vi "ActionVIOnCompile.vi"(8 "error in (no error)":errorcluster, 11 "Device Item Ref in":T3 format="%.0x") -> (0 "error out":errorcluster)   [LabVIEW 2017]
uses:
  <vilib>/NI Veristand/Custom Device API/Custom Device Item Ref.ctl
  Shared/Constants.vi
  <vilib>/NI Veristand/Custom Device API/Get Item Property (I32).vi
  <vilib>/NI Veristand/Custom Device API/Get Item Property (U32).vi
  <vilib>/NI Veristand/Custom Device API/Get Item Property (String).vi
  <vilib>/NI Veristand/Custom Device API/Set Item Property (Variant).vi
  <vilib>/NI Veristand/Custom Device API/Custom Device API.lvlib
  Shared/O2SensorSim_SLSC Shared.lvlib
panel:
  in  "Compiled.Settings 2":T1={"Name"="", "SLSC IP Address"="", "Slot #"=0, "Configuration Data"={"Properties"={"Boolean Properties"=[], "Double Properties"=[], "I32 Properties"=[], "I64 Properties"=[], "String Properties"=[], "U32 Properties"=[], "U64 Properties"=[]}}, "SLSC Set Properties"=[], "SLSC Get Properties"=[], "SLSC Commands"=[], "Username"="admin", "Password"="", "Support Modules"=[]}
  out "Found":bool
  out "support module":T2(array[cluster])
  out "appended array 2":T2(array[cluster]) {"Dev.ProductNumber" format="%.0x"; "Dev.VendorNumber" format="%.0x"}
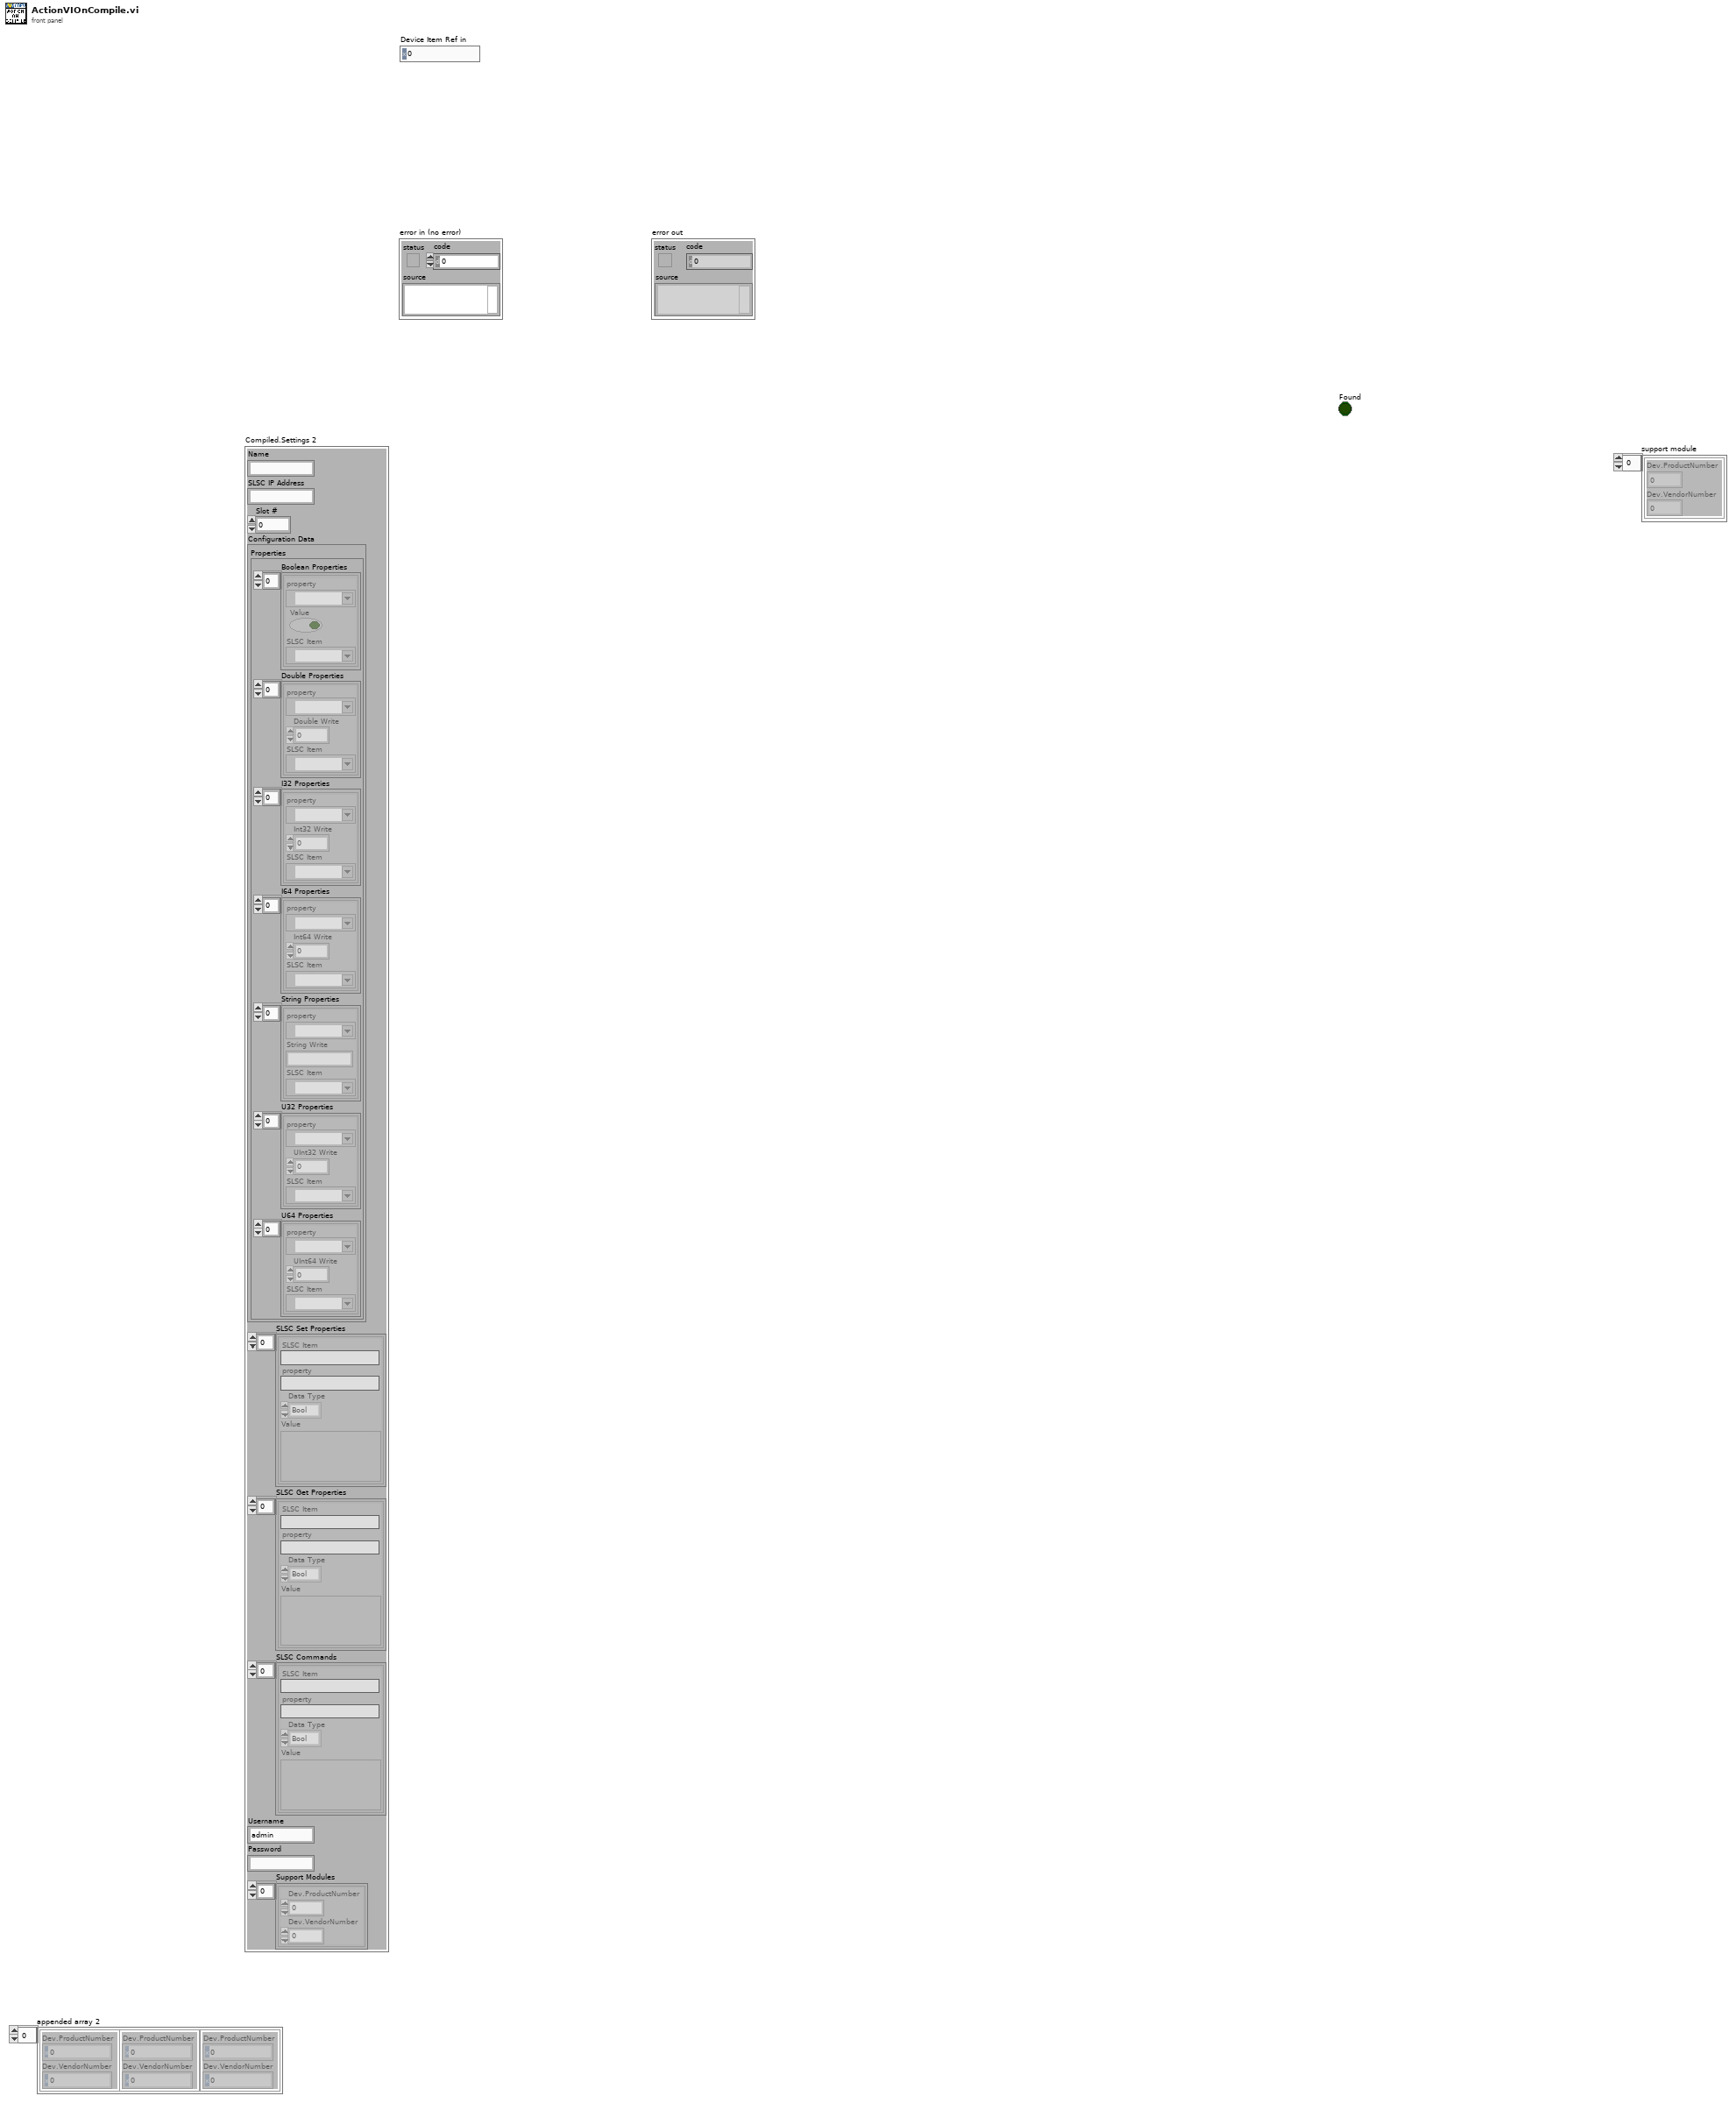
[diagram p1: front panel]
types:
  T1 = cluster{"Name":string, "SLSC IP Address":string, "Slot #":i32, "Configuration Data":cluster{"Properties":cluster{"Boolean Properties":cluster{"property":refnum<k21>, "Value":bool, "SLSC Item":refnum<k21>}[], "Double Properties":cluster{"property":refnum<k21>, "Double Write":dbl, "SLSC Item":refnum<k21>}[], "I32 Properties":cluster{"property":refnum<k21>, "Int32 Write":i32, "SLSC Item":refnum<k21>}[], "I64 Properties":cluster{"property":refnum<k21>, "Int64 Write":i64, "SLSC Item":refnum<k21>}[], "String Properties":cluster{"property":refnum<k21>, "String Write":string, "SLSC Item":refnum<k21>}[], "U32 Properties":cluster{"property":refnum<k21>, "UInt32 Write":u32, "SLSC Item":refnum<k21>}[], "U64 Properties":cluster{"property":refnum<k21>, "UInt64 Write":u64, "SLSC Item":refnum<k21>}[]}}, "SLSC Set Properties":cluster{"SLSC Item":string, "property":string, "Data Type":enum16{"Bool", "Double", "I32", "I64", "String", "U32", "U64", "EnumI32"}, "Value":variant}[], "SLSC Get Properties":cluster{"SLSC Item":string, "property":string, "Data Type":enum16{"Bool", "Double", "I32", "I64", "String", "U32", "U64", "EnumI32"}, "Value":variant}[], "SLSC Commands":cluster{"SLSC Item":string, "property":string, "Data Type":enum16{"Bool", "Double", "I32", "I64", "String", "U32", "U64", "EnumI32"}, "Value":variant}[], "Username":string, "Password":string, "Support Modules":cluster{"Dev.ProductNumber":u32, "Dev.VendorNumber":u32}[]}
  T2 = cluster{"Dev.ProductNumber":u32, "Dev.VendorNumber":u32}[]
  T3 = typedef "Custom Device API.lvlib/Custom Device Item Ref.ctl" = u64
  T4 = cluster{"Dev.ProductNumber":u32, "Dev.VendorNumber":u32}
  T5 = typedef "Custom Device API.lvlib/Custom Device Item Info.ctl" = cluster{"Name":string, "Is Channel":bool, "GUID":string, "Is Waveform":bool}
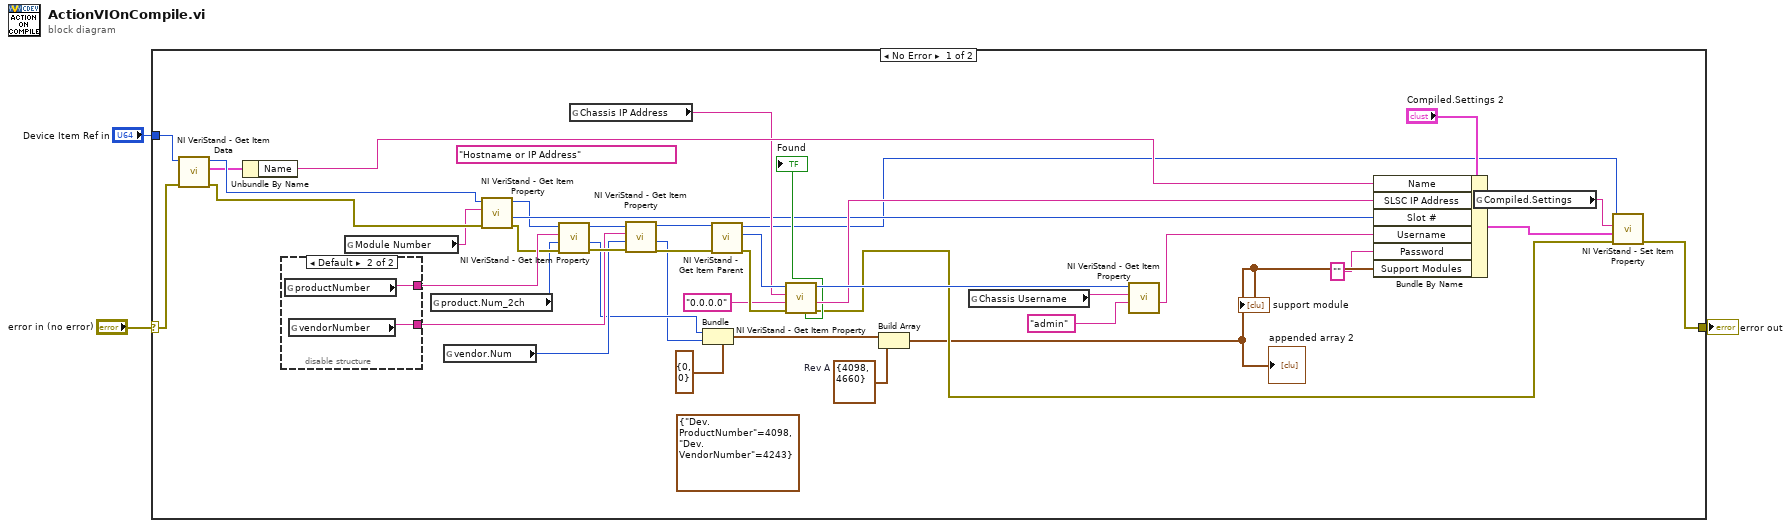
[diagram p0: block diagram]
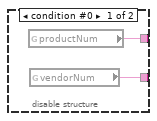
[diagram p2: hidden frame]
diagram:
  n1 = case shown="No Error" "error in (no error)" {
    selector: "error in (no error)" -> [w5 w49]
    tunnel: [w4 w49] -> w2
    tunnel: "Device Item Ref in" -> [w6 _]
    frame No Error {
      (unwired) "Hostname or IP Address" ("Default Value")
      (unwired) T4 {"Dev.ProductNumber"=4098, "Dev.VendorNumber"=4243} ("element")
      w7 = T4 {"Dev.ProductNumber"=4098, "Dev.VendorNumber"=4660}  # Rev A
      n2 = call <vilib>:"NI VeriStand - Get Item Data.vi"("error in (no error)"=w5, "Item Ref in"=w6) -> ("error out"=w41:errorcluster, "Item Info"=w40:T5, "Item Ref out"=w42:T3)  [unwired: 7 out]
      n3 = Unbundle By Name(w40) -> ("Name"=w43:string)
      n4 = disable-structure shown="Default" {
        disable-tunnel: [w46 w48] -> w26
        disable-tunnel: [w45 w47] -> w17
        frame condition #0 {
          n5 = global read "Constants.vi" "productNum"() -> (w46:string)
          n6 = global read "Constants.vi" "vendorNum"() -> (w45:string)
        }
        frame condition #1 (active) {
          n7 = global read "Constants.vi" "productNumber"() -> (w48:string)
          n8 = global read "Constants.vi" "vendorNumber"() -> (w47:string)
        }
      }
      n9 = global read "Constants.vi" "Module Number"() -> (w30:string)
      n10 = global read "Constants.vi" "product.Num_2ch"() -> (w21:i32)
      n11 = global read "Constants.vi" "vendor.Num"() -> (w16:i32)
      n12 = call-poly <vilib>:"NI VeriStand - Get Item Property.vi"("error in (no error)"=w41, "Property Name"=w30, "Item Ref in"=w42) -> ("error out"=w24:errorcluster, "Value"=w31:i32, "Item Ref out"=w25:T3)  [unwired: 5 in, 1 out]
      n13 = call-poly <vilib>:"NI VeriStand - Get Item Property.vi"("error in (no error)"=w24, "Default Value"=w21, "Property Name"=w26, "Item Ref in"=w25) -> ("error out"=w18:errorcluster, "Value"=w13:u32, "Item Ref out"=w20:T3)  [unwired: 4 in, 1 out]
      n14 = global read "Constants.vi" "Chassis IP Address"() -> (w37:string)
      n15 = call-poly <vilib>:"NI VeriStand - Get Item Property.vi"("error in (no error)"=w18, "Default Value"=w16, "Property Name"=w17, "Item Ref in"=w20) -> ("error out"=w19:errorcluster, "Value"=w12:u32, "Item Ref out"=w39:T3)  [unwired: 4 in, 1 out]
      n16 = Bundle(cluster=T4 {"Dev.ProductNumber"=0, "Dev.VendorNumber"=0} ("Product Identification"), "Dev.ProductNumber"=w13, "Dev.VendorNumber"=w12) -> (w14:T4)
      n17 = call <vilib>:"NI VeriStand - Get Item Parent.vi"("error in (no error)"=w19, "Item Ref in"=w39) -> ("error out"=w32:errorcluster, "Parent Ref"=w38:T3, "Item Ref out"=w27:T3)  [unwired: 6 in, 1 out]
      n18 = call-poly <vilib>:"NI VeriStand - Get Item Property.vi"("error in (no error)"=w32, "Default Value"="0.0.0.0", "Property Name"=w37, "Item Ref in"=w38) -> ("error out"=w28:errorcluster, "Value"=w35:string, "Item Ref out"=w36:T3, "Found?"=→"Found":bool)  [unwired: 4 in]
      n19 = Build Array(w14, w7) -> (w15:T2)
      "appended array 2" <- w15
      "support module" <- w15
      n20 = global read "Constants.vi" "Chassis Username"() -> (w23:string)
      n21 = call-poly <vilib>:"NI VeriStand - Get Item Property.vi"("Default Value"="admin", "Property Name"=w23, "Item Ref in"=w36) -> ("Value"=w22:string)  [unwired: 5 in, 3 out]
      n22 = Bundle By Name(cluster="Compiled.Settings 2", "Name"=w43, "SLSC IP Address"=w35, "Slot #"=w31, "Username"=w22, "Password"="", "Support Modules"=w15) -> (w33:T1)
      n23 = global read "Constants.vi" "Compiled.Settings"() -> (w29:string)
      n24 = call-poly <vilib>:"NI VeriStand - Set Item Property.vi"("error in (no error)"=w28, "Value"=w33, "Property Name"=w29, "Item Ref in"=w27) -> ("error out"=w4:errorcluster)  [unwired: 5 in, 2 out]
    }
    frame Error {
    }
  }
  "error out" <- w2
